vi "pll.vi"() -> ()   [LabVIEW 2019]
uses:
  <vilib>/DAQmx/write.llb/DAQmx Write (Analog 1D DBL 1Chan NSamp).vi
  <vilib>/DAQmx/read.llb/DAQmx Read (Counter 1D U32 1Chan NSamp).vi
  <vilib>/Analysis/baseanly.llb/Mean (DBL).vi
  <vilib>/DAQmx/create/channels.llb/DAQmx Create Channel (CI-Count Edges).vi
  <vilib>/DAQmx/configure/timing.llb/DAQmx Timing (Sample Clock).vi
  <vilib>/DAQmx/create/channels.llb/DAQmx Create Channel (AO-Voltage-Basic).vi
  <vilib>/DAQmx/miscellaneous.llb/DAQmx Fill In Error Info.vi
  <vilib>/DAQmx/configure/trigger.llb/DAQmx Start Trigger (Digital Edge).vi
  <vilib>/Analysis/NI_AALBase.lvlib
  <resource>/objmgr/daqmx.rc
panel:
  out "element":u32
  out "SampClk.TimebaseDiv":u32
  out "32bit integer":i32
  out "number of samples written per channel":u32
  out "TotalSampPerChanGenerated":dbl
  out "Numeric":u32
  out "size(s)":i32
  out "mean":dbl format="%0.2f"
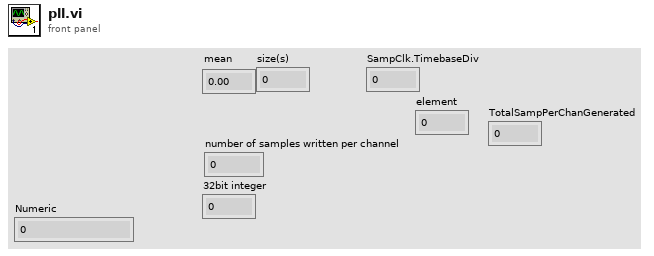
[diagram p1: front panel]
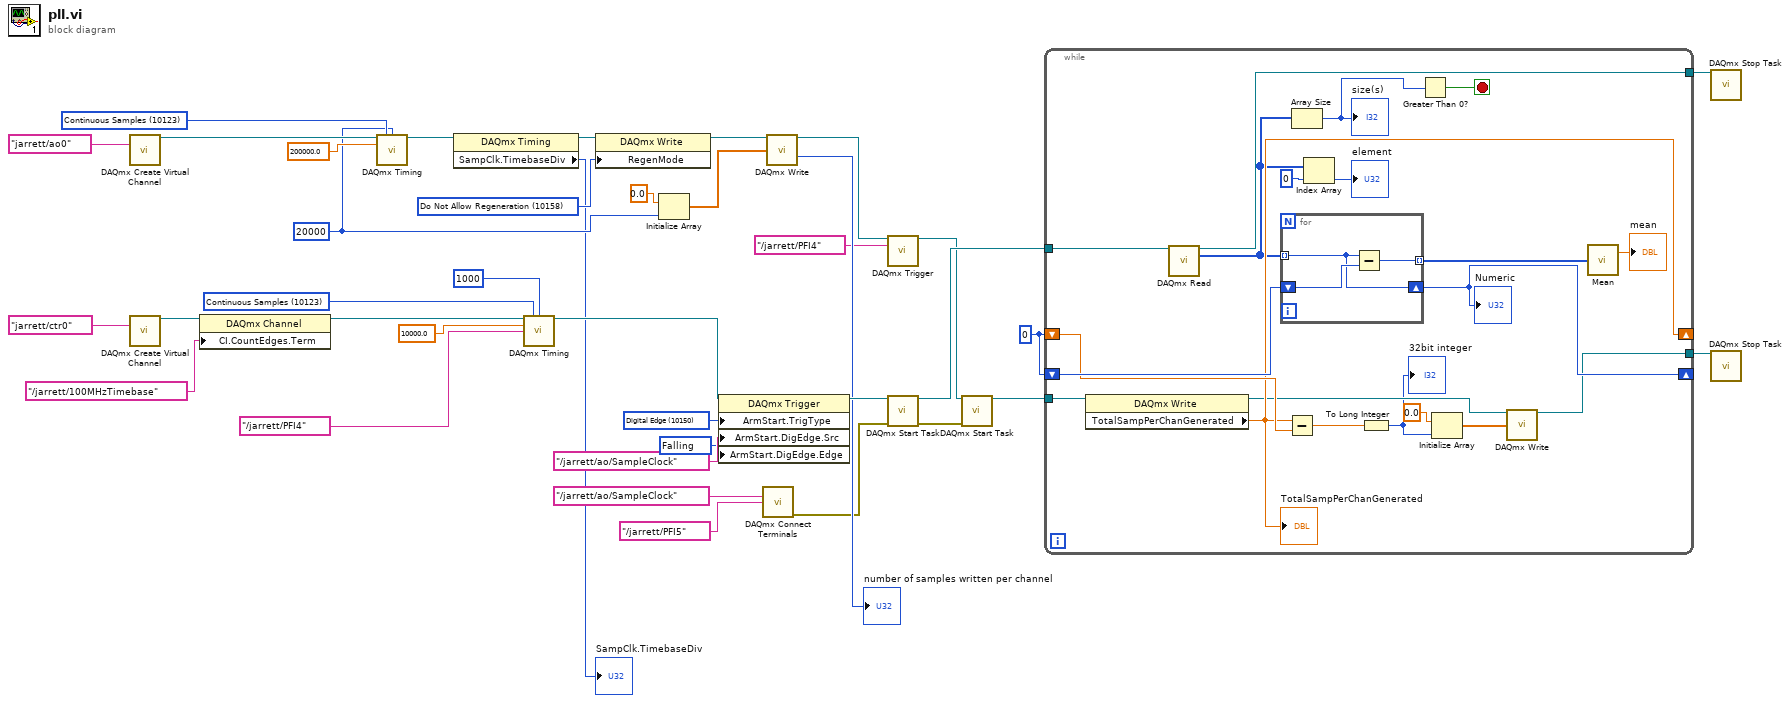
[diagram p0: block diagram]
diagram:
  w1 = 10171 items=["Rising"=10280, "Falling"=10171] ("ArmStart.DigEdge.Edge")
  w14 = 10158 items=["Allow Regeneration"=10097, "Do Not Allow Regeneration"=10158] ("RegenMode")
  w21 = 10150 items=["Digital Edge"=10150, "Time"=15996, "None"=10230] ("ArmStart.TrigType")
  w18 = 20000 ("samples per channel")
  w28 = 10123 items=["Finite Samples"=10178, "Continuous Samples"=10123, "Hardware Timed Single Point"=12522] ("sample mode")
  w17 = 0
  w37 = 10123 items=["Finite Samples"=10178, "Continuous Samples"=10123, "Hardware Timed Single Point"=12522] ("sample mode")
  n1 = call-poly <vilib>:"DAQmx Create Virtual Channel.vi"("physical channels"=tag "jarrett/ao0") -> ("task out"=w29:refnum<k21>)  [unwired: 13 in, 1 out]
  n2 = call-poly <vilib>:"DAQmx Create Virtual Channel.vi"("counter"=tag "jarrett/ctr0") -> ("task out"=w32:refnum<k21>)  [unwired: 13 in, 1 out]
  n3 = property class="DAQmx Channel"(reference=w32, "CI.CountEdges.Term"=tag "/jarrett/100MHzTimebase") -> (reference out=w31:refnum<k21>)  [unwired: 1 in, 1 out]
  n4 = call-poly <vilib>:"DAQmx Timing.vi"("task/channels in"=w29, "sample mode"=w28, "samples per channel"=w18, "rate"=200000.0) -> ("task out"=w8:refnum<k21>)  [unwired: 10 in, 1 out]
  n5 = property class="DAQmx Timing"(reference=w8) -> (reference out=w7:refnum<k21>, "SampClk.TimebaseDiv"=→"SampClk.TimebaseDiv":u32)  [unwired: 1 in, 1 out]
  n6 = call-poly <vilib>:"DAQmx Timing.vi"("task/channels in"=w31, "sample mode"=w37, "samples per channel"=1000, "rate"=10000.0, "source"=tag "/jarrett/PFI4") -> ("task out"=w16:refnum<k21>)  [unwired: 9 in, 1 out]
  n7 = property class="DAQmx Write"(reference=w7, "RegenMode"=w14) -> (reference out=w13:refnum<k21>)  [unwired: 1 in, 1 out]
  n8 = Initialize Array(0.0 ("element"), w18) -> (w25:dbl[])
  n9 = property class="DAQmx Trigger"(reference=w16, "ArmStart.TrigType"=w21, "ArmStart.DigEdge.Src"=tag "/jarrett/ao/SampleClock", "ArmStart.DigEdge.Edge"=w1) -> (reference out=w15:refnum<k21>)  [unwired: 1 in, 1 out]
  n10 = call <vilib>:"DAQmx Connect Terminals.vi"("source terminal"=tag "/jarrett/ao/SampleClock", "destination terminal"=tag "/jarrett/PFI5") -> ("error out"=w3:errorcluster)  [unwired: 13 in]
  n11 = call-poly <vilib>:"DAQmx Write.vi"("task/channels in"=w13, "data"=w25) -> ("task out"=w12:refnum<k21>, "number of samples written per channel"=→"number of samples written per channel":u32)  [unwired: 11 in, 1 out]
  n12 = call-poly <vilib>:"DAQmx Trigger.vi"("task/channels in"=w12, "source"=tag "/jarrett/PFI4") -> ("task out"=w10:refnum<k21>)  [unwired: 12 in, 1 out]
  n13 = call <vilib>:"DAQmx Start Task.vi"("task/channels in"=w15, "error in"=w3) -> ("task out"=w34:refnum<k21>, "error out"=w2:errorcluster)  [unwired: 12 in]
  n14 = call <vilib>:"DAQmx Start Task.vi"("task/channels in"=w10, "error in"=w2) -> ("task out"=w24:refnum<k21>)  [unwired: 12 in, 1 out]
  n15 = while {
    tunnel: w34 -> [w58]
    tunnel: [w57] -> w33
    shift-right: [w55] -> _
    shift-left: w17 -> [w56]
    shift-right: [w51] -> _
    shift-left: w17 -> [w52]
    tunnel: w24 -> [w46]
    tunnel: [w47] -> w23
    stop <- w42 stop-if-true
    n16 = property class="DAQmx Write"(reference=w46) -> (reference out=w45:refnum<k21>, "TotalSampPerChanGenerated"=w51:dbl)  [unwired: 1 in, 1 out]
    "TotalSampPerChanGenerated" <- w51
    n17 = call-poly <vilib>:"DAQmx Read.vi"("task/channels in"=w58) -> ("task out"=w57:refnum<k21>, "data"=w41:u32[])  [unwired: 12 in, 1 out]
    n18 = for {
      tunnel: w41 -> [w60] mode=indexing
      shift-right: [w60] -> w55
      shift-left: w56 -> [w61]
      tunnel: [w59] -> w54 mode=indexing
      n19 = Subtract(x=w60, y=w61) -> (x-y=w59:u32)
    }
    "Numeric" <- w55
    n20 = Subtract(x=w51, y=w52) -> (x-y=w50:dbl)
    n21 = Array Size(array=w41) -> (size(s)=w43:i32)
    "size(s)" <- w43
    n22 = Index Array(array=w41, index=0) -> (element=→"element":u32)
    n23 = To Long Integer(number=w50) -> (32bit integer=w44:i32)
    "32bit integer" <- w44
    n24 = Greater Than 0?(x=w43) -> (x > 0?=w42:bool)
    n25 = Initialize Array(0.0 ("element"), w44) -> (w48:dbl[])
    n26 = call-poly <vilib>:"DAQmx Write.vi"("task/channels in"=w45, "data"=w48) -> ("task out"=w47:refnum<k21>)  [unwired: 11 in, 2 out]
    n27 = call-poly <vilib>:"Mean.vi"("X"=w54) -> ("mean"=→"mean":dbl)  [unwired: 1 out]
  }
  n28 = call <vilib>:"DAQmx Stop Task.vi"("task/channels in"=w33) -> ()  [unwired: 13 in, 2 out]
  n29 = call <vilib>:"DAQmx Stop Task.vi"("task/channels in"=w23) -> ()  [unwired: 13 in, 2 out]
